vi "Merge text metadata.vi"(11 "Input metadata text array":string[](array[string])) -> (3 "Merged metadata text":string)   [LabVIEW 2015]
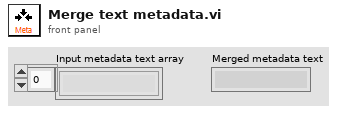
[diagram p1: front panel]
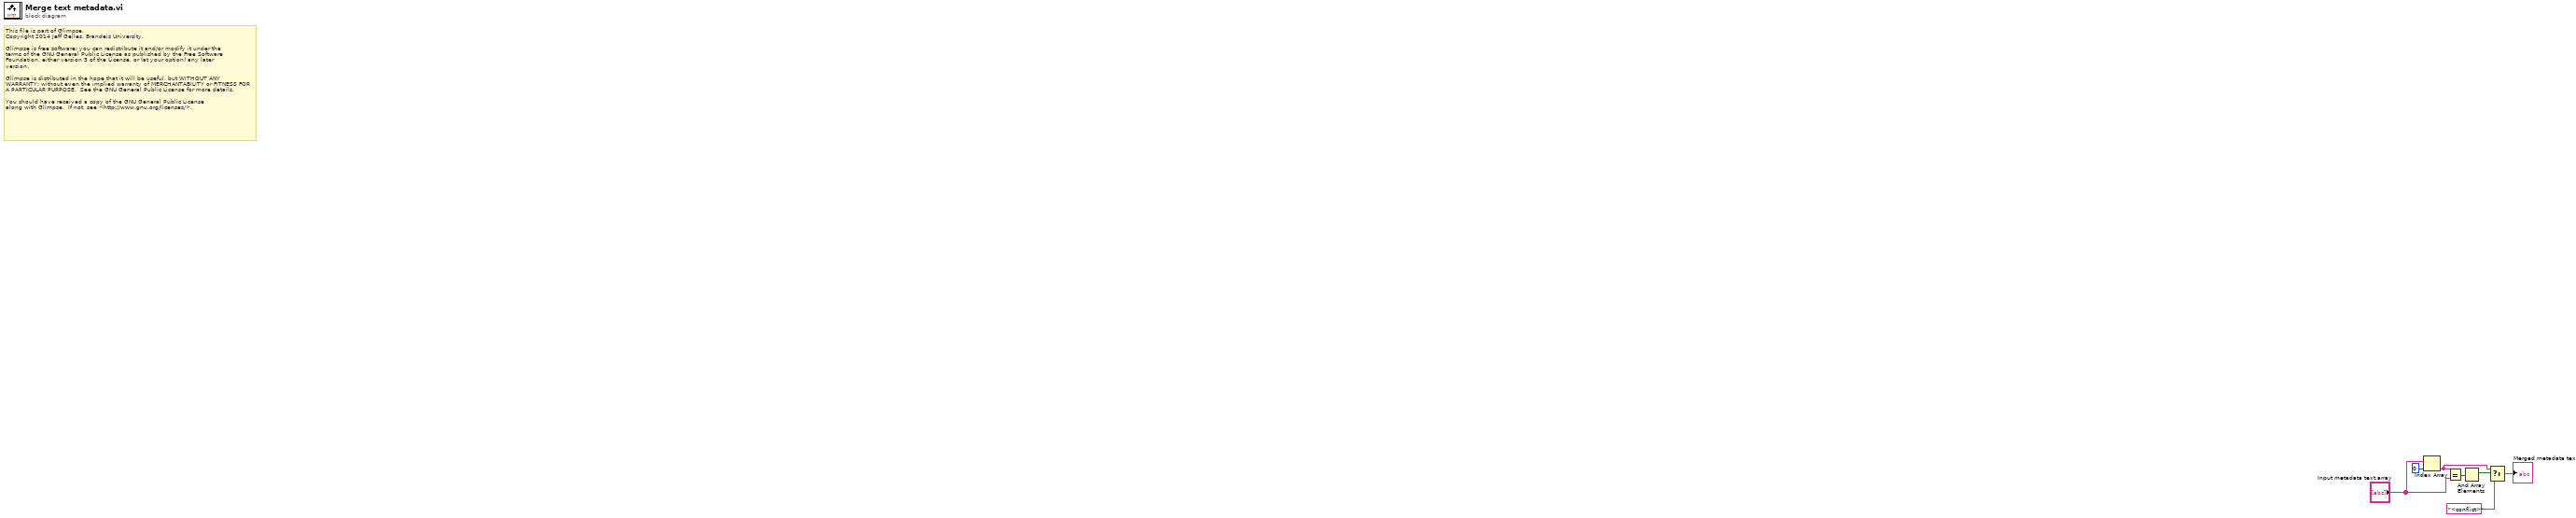
[diagram p0: block diagram]
diagram:
  # "This file is part of Glimpse. \nCopyright 2014 Jeff Gelles, Brandeis University.    \n\nGlimpse is free software: you can redistribute it and/or modify it under the \nterms of the GNU General Public License as published by the Free Software \nFoundation, either version 3 of the License, or (at your option) any later \nversion.\n\nGlimpse is distributed in the hope that it will be useful, but WITHOUT ANY \nWARRANTY; without even the implied warranty of MERCHANTABILITY or FITNESS FOR \nA PARTICULAR PURPOSE.  See the GNU General Public License for more details.\n\nYou should have received a copy of the GNU General Public License\nalong with Glimpse.  If not, see <http://www.gnu.org/licenses/>."
  n1 = Index Array(array="Input metadata text array", index=0) -> (element=w5:string)
  n2 = Equal?(x=w5, y="Input metadata text array") -> (x = y?=w4:bool[])
  n3 = And Array Elements(Boolean array=w4) -> (logical AND=w1:bool)
  n4 = Select(t=w5, s=w1, f="<conflict>") -> (s? t:f=→"Merged metadata text":string)
